vi "Trainer.vi"(0 "svm_parameter":T1={"svm_type"=0, "kernel_type"=2, "degree"=3, "gamma"=0.0, "coef0"=0.0, "cache_size"=40.0, "epsilon"=0.001, "C"=1000.0, "nr_weight"=0, "weight_label"=[1, -1], "Weight (C of class i)"=[1.0, 1.0], "nu"=0.5, "p"=0.1, "Shrinking"=1, "probability"=0} {"p" format="%.4f"; "nu" format="%.4f"; "Weight (C of class i)" format="%.2f"; "C" format="%.2f"; "epsilon" format="%.4f"; "cache_size" format="%.2f"; "coef0" format="%.2f"; "gamma" format="%.5f"; "kernel_type" items=["Linear", "Poly", "RBF", "Sigmoid"]; "svm_type" items=["C-SVC", "Nu-SVC", "One-class SVM", "epsilon-SVR", "nu-SVR"]}, 1 "attributes":dbl[][](array[numeric])=[[23.09, 19.84, 4.59, 25.8, 6.17, 14.76, 36.15, 12.17, 42.58, 21.6, 12.72, 57.75, 68.88, 48.44, 45.21, 30.69, 38.2, 29.51, 22.95, 21.5, 33.14, 42.25, 38.67, 23.8, 58.56, 31.73, 31.61, 41.07, 49.29, 30.54, 55.77, 43.06, 58.33, 16.56, 24.23, 53.03, 40.72, 27.72, 19.85, 17.03, 28.75, 48.31, 37.15, 33.6, 47.43, 22.97, 35.18, 43.94, 79.07, 41.95, 39.05, 23.05, 34.09, 35.16, 48.03, 19.84, 29.81, 28.05, 23.48, 27.6, 30.39], [128.18, 177.72, 179.89, 110.47, 153.07, 133.9, 144.67, 121.74, -130.24, 117.17, 154.56, 89.5, 33.24, 84.79, 46.55, 35.19, 25.36, 53.48, 65.49, 75.03, 59.52, 26.36, 49.83, 39.81, 46.47, 40.03, 52.8, 34.68, 29.83, 58.96, 42.88, 52.84, 113.87, 68.51, 43.86, 42.39, 110.71, 43.27, 16.42, 47.03, 19.33, 34.31, 56.87, 26.65, 60.68, 49.63, 38.39, 51.34, 35.82, 69.25, 72.56, 24.77, 71.56, 74.49, 27.67, 65.55, 28.89, 30.13, 38.62, 17.79, 83.64], [115.25, -83.36, -179.7, 96.59, 120.47, 121.21, 113.01, -147.61, -155.44, 64.08, 35.72, 40.39, 22.52, 46.17, 38.62, 18.42, -18.15, 40.69, 53.18, 54.05, 37.03, 12.7, 36.99, 28.34, 22.69, 30.36, 32.48, 19.19, 15.03, 42.0, 31.05, 39.63, 45.36, 36.55, 30.74, 40.25, 52.91, 27.46, 0.72, 40.32, 14.25, 26.44, 31.53, 14.63, 43.75, 36.38, 27.26, 43.3, 26.22, 54.18, 48.12, 8.01, 59.72, 34.83, 22.66, 40.9, -19.63, 22.81, 11.72, 2.11, 33.05], [8.61, 254.8, 359.58, 9.69, 17.37, 12.7, 16.68, 268.48, 21.09, 42.87, 111.42, 37.4, 8.65, 38.62, 7.67, 16.77, 38.34, 8.3, 6.78, 12.72, 22.49, 12.96, 12.84, 8.89, 23.2, 7.12, 14.38, 15.49, 6.57, 16.23, 11.14, 6.12, 68.51, 17.16, 12.34, 1.83, 57.35, 6.63, 9.22, 5.63, 5.04, 5.29, 25.34, 8.56, 13.07, 13.25, 8.18, 5.65, 7.64, 7.55, 19.78, 14.34, 6.28, 23.07, 4.85, 13.32, 15.98, 6.36, 23.4, 8.38, 50.59], [39.81, 99.46, 106.7, 11.31, 50.19, 45.0, 59.04, 141.34, 135.0, 35.54, 48.81, -51.34, -59.04, -9.46, -51.34, -51.34, -68.2, -45.0, -33.69, -18.43, -51.34, -63.43, -38.66, -59.04, -51.34, -50.19, -45.0, -51.34, -63.43, -45.0, -51.34, -51.34, -33.69, -29.05, -51.34, -51.34, -33.69, -45.0, -74.05, -45.0, -71.57, -51.34, -9.46, -56.31, -50.19, -33.69, -51.34, -45.0, -56.31, -38.66, -38.66, -63.43, -26.57, -51.34, -63.43, -38.66, -68.2, -18.43, 0.0, -71.57, -50.19], [-45.0, 11.31, 29.74, -38.66, 26.57, 15.95, 33.69, 26.57, 116.57, 26.57, -40.6, -66.8, -71.57, -56.31, -63.43, -63.43, -111.8, -56.31, -45.0, -56.31, -63.43, -71.57, -51.34, -66.8, -63.43, -56.31, -59.04, -63.43, -71.57, -51.34, -66.8, -51.34, -38.66, -56.31, -63.43, -51.34, -45.0, -63.43, -99.46, -51.34, -81.87, -59.04, -59.04, -71.57, -56.31, -51.34, -63.43, -51.34, -63.43, -56.31, -63.43, -74.05, -38.66, -66.8, -71.57, -51.34, -111.8, -71.57, -30.96, -81.87, -56.31], [54.46, 88.15, 76.95, 49.97, 16.5, 29.05, 14.04, 114.78, 11.31, 7.13, 88.97, 15.46, 8.13, 46.85, 7.13, 12.09, 33.11, 11.31, 11.31, 32.91, 12.09, 8.13, 12.68, 7.77, 12.09, 6.12, 11.31, 12.09, 8.13, 6.34, 15.46, 0.0, 4.97, 11.55, 12.09, 0.0, 11.31, 18.43, 18.92, 6.34, 10.3, 7.7, 49.57, 8.13, 6.12, 11.31, 12.09, 6.34, 7.13, 12.68, 17.65, 8.13, 12.09, 15.46, 8.13, 6.34, 22.62, 40.6, 30.96, 10.3, 6.12], [49.71, 88.81, 52.6, 28.06, 41.64, 35.7, 24.8, 16.16, 14.78, 27.82, 84.63, 24.25, 17.55, 23.95, 16.16, 17.55, 19.67, 16.16, 28.14, 43.07, 27.6, 7.67, 14.93, 35.7, 16.16, 11.98, 16.16, 16.16, 7.67, 13.36, 24.25, 0.0, 16.16, 28.19, 16.16, 0.0, 16.16, 21.03, 23.95, 13.36, 23.95, 11.44, 14.93, 10.06, 11.98, 16.16, 17.55, 13.36, 10.06, 28.28, 28.14, 25.82, 16.16, 33.18, 7.67, 13.36, 7.7, 11.44, 24.8, 19.77, 11.98], [0.28, 1.58, 0.18, 0.78, 0.35, 0.67, 0.38, 1.55, 0.69, 0.7, 1.56, 0.13, 0.13, 0.75, 0.21, 0.39, 0.91, 0.26, 0.18, 0.23, 0.44, 0.28, 0.15, 0.28, 0.16, 0.12, 1.17, 0.43, 0.42, 0.1, 0.3, 0.13, 0.12, 0.15, 0.15, 0.14, 0.23, 0.4, 0.59, 0.31, 0.83, 0.14, 0.64, 0.47, 0.2, 0.65, 0.21, 0.4, 0.32, 0.29, 0.33, 0.58, 0.12, 0.26, 0.38, 0.11, 0.11, 0.68, 0.35, 0.92, 0.7]], 2 "Lables":dbl[](array[numeric])=[1.0, 1.0, 1.0, 1.0, 1.0, 1.0, 1.0, 1.0, 1.0, 1.0, 1.0, -1.0, -1.0, -1.0, -1.0, -1.0, -1.0, -1.0, -1.0, -1.0, -1.0, -1.0, -1.0, -1.0, -1.0, -1.0, -1.0, -1.0, -1.0, -1.0, -1.0, -1.0, -1.0, -1.0, -1.0, -1.0, -1.0, -1.0, -1.0, -1.0, -1.0, -1.0, -1.0, -1.0, -1.0, -1.0, -1.0, -1.0, -1.0, -1.0, -1.0, -1.0, -1.0, -1.0, -1.0, -1.0, -1.0, -1.0, -1.0, -1.0, -1.0], 3 "ModelFileName":string="C:\\\\WORK\\\\tempModel") -> ()   [LabVIEW 2014]
doc: "This is the trainer module for LIBSVM interface developed by kwkim@kriss.re.kr."
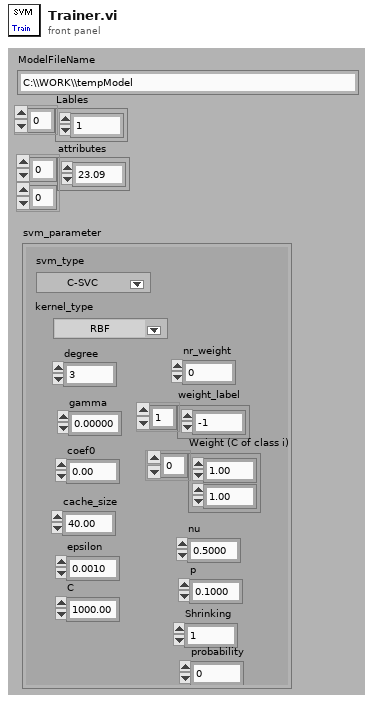
[diagram p1: front panel]
types:
  T1 = cluster{"svm_type":i16, "kernel_type":i16, "degree":i16, "gamma":dbl, "coef0":dbl, "cache_size":dbl, "epsilon":dbl, "C":dbl, "nr_weight":i16, "weight_label":i16[], "Weight (C of class i)":dbl[], "nu":dbl, "p":dbl, "Shrinking":i16, "probability":i16}
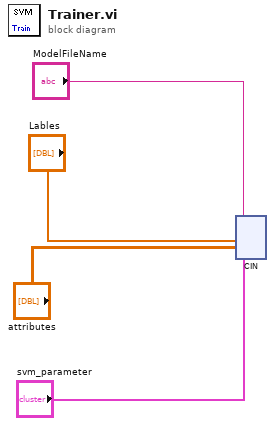
[diagram p0: block diagram]
diagram:
  n1 = cin("ModelFileName", "Lables", "attributes", "svm_parameter") -> ()  [unwired: 4 in]
